vi "AnalogControl.vi"(0 "controller in":refnum<k24>, 1 "analog input":i32, 2 "offset value":dbl, 3 "speed value":dbl, 5 "axis name":string, 7 "on/off":i32(ring) items=["Off", "On"], 11 "error in (no error)":errorcluster, 12 "scale factor":dbl=1.0, 13 "return immediately":bool) -> (4 "controller out":refnum<k24>, 15 "error out":errorcluster)   [LabVIEW 2010]
uses:
  c:/aerotech/controller/5.xx.xxx/ensemble/pc/labview/2010/bin/Aerotech.Ensemble.dll
  bin/Aerotech.Ensemble.dll
  c:/aerotech/controller/5.xx.xxx/ensemble/pc/labview/2010/bin/Aerotech.Ensemble.LabVIEW.dll
  bin/Aerotech.Ensemble.LabVIEW.dll
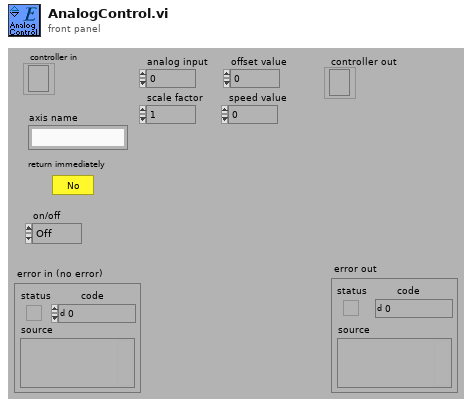
[diagram p1: front panel]
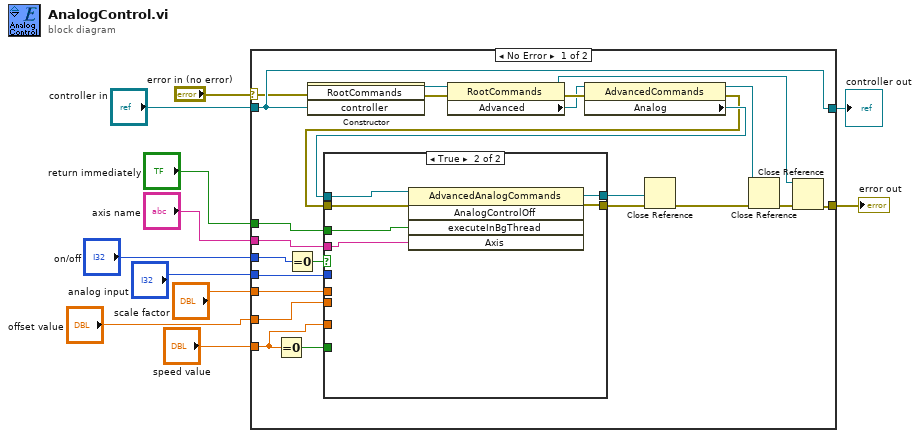
[diagram p0: block diagram]
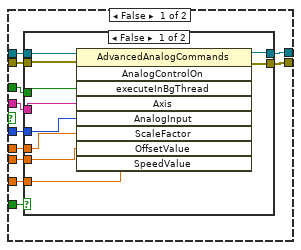
[diagram p2: hidden frame]
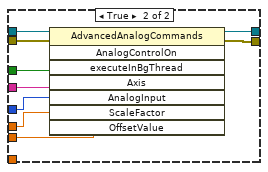
[diagram p3: hidden frame]
diagram:
  n1 = case shown="No Error" "error in (no error)" {
    selector: "error in (no error)" -> [w14 w73]
    tunnel: [w25 w73] -> w10
    tunnel: "controller in" -> [w20 w72]
    tunnel: "return immediately" -> [w29 _]
    tunnel: "axis name" -> [w28 _]
    tunnel: "on/off" -> [w13 _]
    tunnel: [w20 w72] -> w5
    tunnel: "analog input" -> [w19 _]
    tunnel: "scale factor" -> [w18 _]
    tunnel: "offset value" -> [w17 _]
    tunnel: "speed value" -> [w15 _]
    frame No Error {
      n2 = Equal To 0?(x=w15) -> (x = 0?=w16:bool)
      n3 = Equal To 0?(x=w13) -> (x = 0?=w12:bool)
      n4 = constructor class="RootCommands"(error in=w14, "controller"=w20) -> (reference out=w35:refnum<k24>, error out=w34:errorcluster)  [unwired: 2 in, 2 out]
      n5 = property class="RootCommands"(reference=w35, error in=w34) -> (reference out=w22:refnum<k24>, error out=w33:errorcluster, "Advanced"=w32:refnum<k24>)
      n6 = property class="AdvancedCommands"(reference=w32, error in=w33) -> (reference out=w23:refnum<k24>, error out=w30:errorcluster, "Analog"=w31:refnum<k24>)
      n7 = case shown="True" w12 {
        tunnel: w31 -> [w46 w70]
        tunnel: w30 -> [w45 w71]
        tunnel: w29 -> [w44 w67]
        tunnel: w28 -> [w43 w66]
        tunnel: [w42 w68] -> w27
        tunnel: [w41 w69] -> w26
        tunnel: w19 -> [w40 _]
        tunnel: w18 -> [w39 _]
        tunnel: w17 -> [w38 _]
        tunnel: w16 -> [w37 _]
        tunnel: w15 -> [w36 _]
        frame False {
          n8 = case shown="False" w37 {
            tunnel: w46 -> [w56 w65]
            tunnel: w45 -> [w55 w64]
            tunnel: w44 -> [w54 w63]
            tunnel: w43 -> [w53 w62]
            tunnel: [w52 w61] -> w42
            tunnel: [w51 w60] -> w41
            tunnel: w40 -> [w47 w59]
            tunnel: w39 -> [w48 w58]
            tunnel: w38 -> [w49 w57]
            tunnel: w36 -> [w50 _]
            frame False {
              n9 = invoke class="AdvancedAnalogCommands" method="AnalogControlOn"(reference=w56, error in=w55, "executeInBgThread"=w54, "Axis"=w53, "AnalogInput"=w47, "ScaleFactor"=w48, "OffsetValue"=w49, "SpeedValue"=w50) -> (reference out=w51:refnum<k24>, error out=w52:errorcluster)  [unwired: 1 in, 7 out]
            }
            frame True {
              n10 = invoke class="AdvancedAnalogCommands" method="AnalogControlOn"(reference=w65, error in=w64, "executeInBgThread"=w63, "Axis"=w62, "AnalogInput"=w59, "ScaleFactor"=w58, "OffsetValue"=w57) -> (reference out=w60:refnum<k24>, error out=w61:errorcluster)  [unwired: 1 in, 6 out]
            }
          }
        }
        frame True {
          n11 = invoke class="AdvancedAnalogCommands" method="AnalogControlOff"(reference=w70, error in=w71, "executeInBgThread"=w67, "Axis"=w66) -> (reference out=w69:refnum<k24>, error out=w68:errorcluster)  [unwired: 1 in, 3 out]
        }
      }
      n12 = Close Reference(reference=w26, error in (no error)=w27) -> (error out=w21:errorcluster)
      n13 = Close Reference(reference=w23, error in (no error)=w21) -> (error out=w24:errorcluster)
      n14 = Close Reference(reference=w22, error in (no error)=w24) -> (error out=w25:errorcluster)
    }
    frame Error {
    }
  }
  "error out" <- w10
  "controller out" <- w5
